vi "Dequeue Logs Element.vi"(8 "Error In":errorcluster, 9 "Timeout":i32=-1, 11 "EventLog in":refnum<class "LogsAbstract.lvclass">) -> (0 "Error Out":errorcluster, 1 "Timed out?":bool, 3 "EventLog out":refnum<class "LogsAbstract.lvclass">)   [LabVIEW 2019, in "LogsAbstract.lvlib" / "LogsAbstract.lvclass"]
uses:
  LogsAbstract.lvclass
  Classes/Event/Event.lvclass
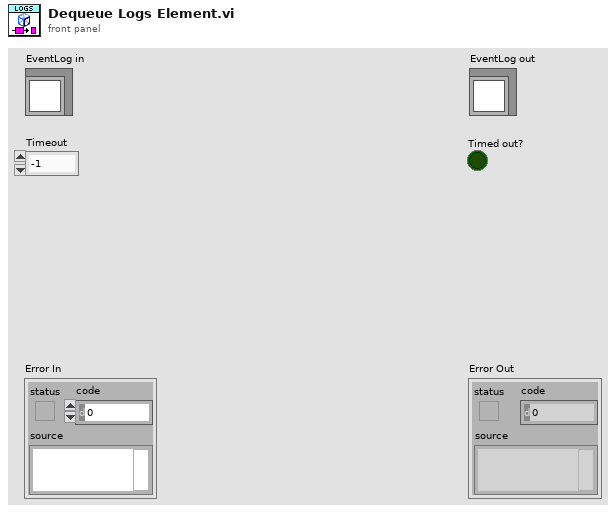
[diagram p1: front panel]
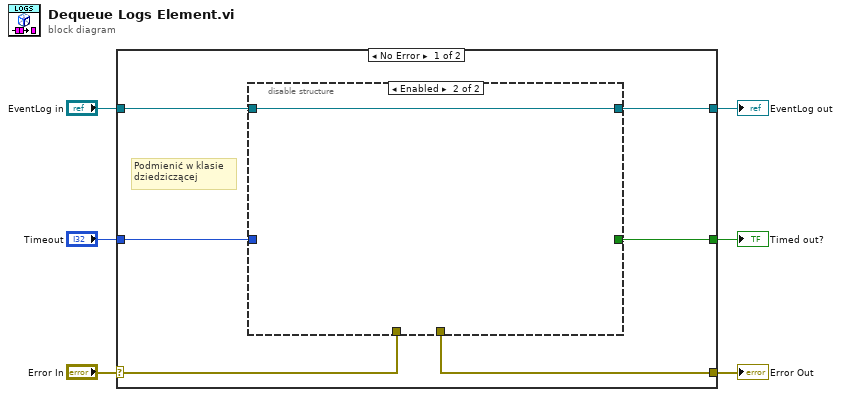
[diagram p0: block diagram]
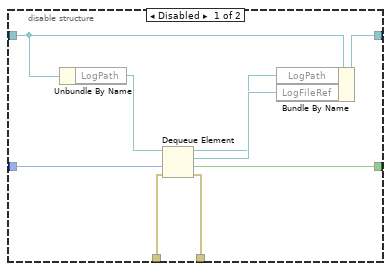
[diagram p2: hidden frame]
diagram:
  n1 = case shown="No Error" "Error In" {
    selector: "Error In" -> [w11 w24]
    tunnel: [w10 w24] -> w5
    tunnel: [w9 w23] -> w3
    tunnel: "EventLog in" -> [w12 w23]
    tunnel: [w8 _] -> w2
    tunnel: "Timeout" -> [w7 _]
    frame No Error {
      # "Podmienić w klasie\ndziedziczącej"
      n2 = disable-structure shown="Enabled" {
        disable-tunnel: w12 -> [w21 w22]
        disable-tunnel: w11 -> [w19 _]
        disable-tunnel: [w18 _] -> w10
        disable-tunnel: [w17 w22] -> w9
        disable-tunnel: [w14 _] -> w8
        disable-tunnel: w7 -> [w13 _]
        frame Disabled {
          n3 = Unbundle By Name(w21) -> ("LogPath"=w20:path)
          n4 = Dequeue Element(queue=w20, timeout in ms (-1)=w13, error in (no error)=w19) -> (queue out=w15:refnum<queue>, element=w16:refnum<class "Event.lvclass">, timed out?=w14:bool, error out=w18:errorcluster)
          n5 = Bundle By Name(cluster=w21, "LogPath"=w15, "LogFileRef"=w16) -> (w17:refnum<class "LogsAbstract.lvclass">)
        }
        frame Enabled {
        }
      }
    }
    frame Error {
    }
  }
  "Error Out" <- w5
  "EventLog out" <- w3
  "Timed out?" <- w2
